vi "VariableRateTest.vi"() -> ()   [LabVIEW 2015]
uses:
  <vilib>/Platform/TimedLoop/XDataNode/timing_clust.ctl
  <vilib>/Platform/TimedLoop/XDataNode/nitl_modes.ctl
  <vilib>/Platform/TimedLoop/XDataNode/wakeup.ctl
  <vilib>/rvi/Emulation/niFpgaGetClockAttributes.vi
  <vilib>/rvi/Emulation/niFpgaSctlEmulationGetInTimedLoop.vi
  <vilib>/rvi/Emulation/niFpgaEmulationReportErrorSimple.vi
  TickTocks/Tock1.vi
  <vilib>/rvi/Emulation/niFpgaCriticalErrorInLSC.vi
  TickTocks/Tick1.vi
  TickTocks/Tock0.vi
  TickTocks/Tick0.vi
  <vilib>/platform/TimedLoop/XDataNode/XDataNode.xnode
  <vilib>/Platform/TimedLoop/XDataNode/XDNodeRunTimeDep.lvlib
  Timers.lvlib
panel:
  in  "tocks_bottom":u32
  in  "ticks_top":u32
  out "MaxTimes":u32[](array[numeric])
  out "Times":u32[](array[numeric])
  in  "resetMaxTime":bool
  in  "sctl_ticks_bottom":u16
  in  "sctl_ticks_top":u16
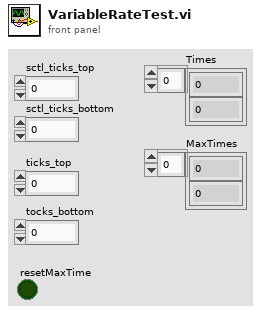
[diagram p1: front panel]
types:
  T1 = typedef "Timers.lvlib/TimerRegisters.ctl" = cluster{"Tick0":refnum<k21>, "Tock0":refnum<k21>, "Tick1":refnum<k21>, "Tock1":refnum<k21>, "Tick2":refnum<k21>, "Tock2":refnum<k21>, "Tick3":refnum<k21>, "Tock3":refnum<k21>, "Tick4":refnum<k21>, "Tock4":refnum<k21>, "Tick5":refnum<k21>, "Tock5":refnum<k21>, "Tick6":refnum<k21>, "Tock6":refnum<k21>, "Tick7":refnum<k21>, "Tock7":refnum<k21>}
  T2 = typedef "XDNodeRunTimeDep.lvlib/timing_clust.ctl" = cluster{"Expected End [f-1]":u64, "Actual End [f-1]":u64, "Finished Late? [f-1]":bool, "Expected End [i-1]":u64, "Actual End [i-1]":u64, "Finished Late? [i-1]":bool, "Expected Start [i]":u64, "Actual Start [i]":u64, "Expected Start [f]":u64, "Actual Start [f]":u64, "Source Name":string, "Structure Name":string, "Period":i64, "Deadline":i64, "Offset":i64, "Start":i64, "Priority":i32, "Timeout":i32, "Mode":T3, "Wakeup Reason":T4, "Error":errorcluster, "Source Type":string, "Secondary Source Type":string, "Global End Time":u64, "Global Start Time":u64, "Frame Duration":u64, "Iteration Duration":u64, "Assigned CPU":i32, "I/O Scan Engine Mode":u32}
  T3 = typedef "XDNodeRunTimeDep.lvlib/nitl_modes.ctl" = enum32{"No Change", "Process missed periods, maintain original phase", "Discard missed periods, maintain original phase", "Process missed periods, ignore original phase", "Discard missed periods, ignore original phase"}
  T4 = typedef "XDNodeRunTimeDep.lvlib/wakeup.ctl" = enum32{"Normal", "Aborted", "Asynchronous wakeup", "Timing source error", "Timed loop error", "Timeout"}
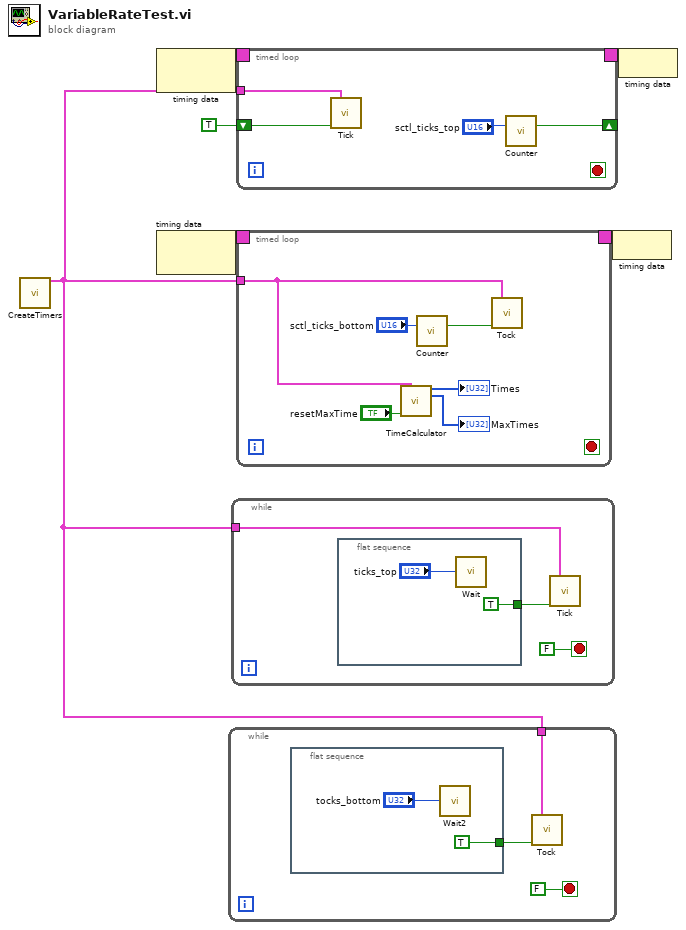
[diagram p0: block diagram]
diagram:
  n1 = call "CreateTimers.vi"() -> ("TimerRegisters"=w2:T1)  [unwired: 15 in]
  n2 = node-c288() -> (w6:T2)  [unwired: 1 in]
  n3 = node-c288() -> (w4:T2)  [unwired: 1 in]
  n4 = while {
    tunnel: w2 -> [w7]
    stop <- FALSE stop-if-true
    n5 = flat-sequence {
      tunnel: [TRUE] -> w8
      frame #0 {
        n6 = call "Wait2"("Count(Ticks)"="tocks_bottom") -> ()  [unwired: 1 out]
      }
    }
    n7 = call-poly "Tock.vi"("TimerRegisters"=w7, "valid input"=w8) -> ()  [unwired: 13 in, 1 out]
  }
  n8 = while {
    tunnel: w2 -> [w13]
    stop <- FALSE stop-if-true
    n9 = flat-sequence {
      tunnel: [TRUE ("valid input")] -> w12
      frame #0 {
        n10 = call "Wait"("Count(Ticks)"="ticks_top") -> ()  [unwired: 1 out]
      }
    }
    n11 = call-poly "Tick.vi"("TimerRegisters"=w13, "valid input"=w12) -> ()  [unwired: 13 in, 1 out]
  }
  n12 = timed-loop {
    timing: w6 -> [_]
    timing-out: [_] -> w5
    tunnel: w2 -> [w20]
    shift-right: [w18] -> _
    shift-left: TRUE ("ding") -> [w17]
    stop <- _ stop-if-true
    n13 = call-poly "Tick.vi"("TimerRegisters"=w20, "valid input"=w17) -> ()  [unwired: 13 in, 1 out]
    n14 = call "Counter.vi"("ticks"="sctl_ticks_top") -> ("ding"=w18:bool)  [unwired: 14 in]
  }
  n15 = timed-loop {
    timing: w4 -> [_]
    timing-out: [_] -> w3
    tunnel: w2 -> [w26]
    stop <- _ stop-if-true
    n16 = call "TimeCalculator.vi"("TimerRegisters"=w26, "resetMaxTime"="resetMaxTime") -> ("Times"=→"Times":u32[], "MaxTimes"=→"MaxTimes":u32[])  [unwired: 12 in]
    n17 = call "Counter.vi"("ticks"="sctl_ticks_bottom") -> ("ding"=w27:bool)  [unwired: 14 in]
    n18 = call-poly "Tock.vi"("TimerRegisters"=w26, "valid input"=w27) -> ()  [unwired: 13 in, 1 out]
  }
  n19 = node-c288(w3) -> ()
  n20 = node-c288(w5) -> ()
